vi "drawing fun.vi"() -> ()   [LabVIEW 2009]
panel:
  in  "stop":bool
  out "point":cluster{"x":i16, "y":i16}
  in  "color":u32(colorbox)
  in  "pen":T1={"Width"=1, "Style"=enum."Solid"}
  out "Picture":picture
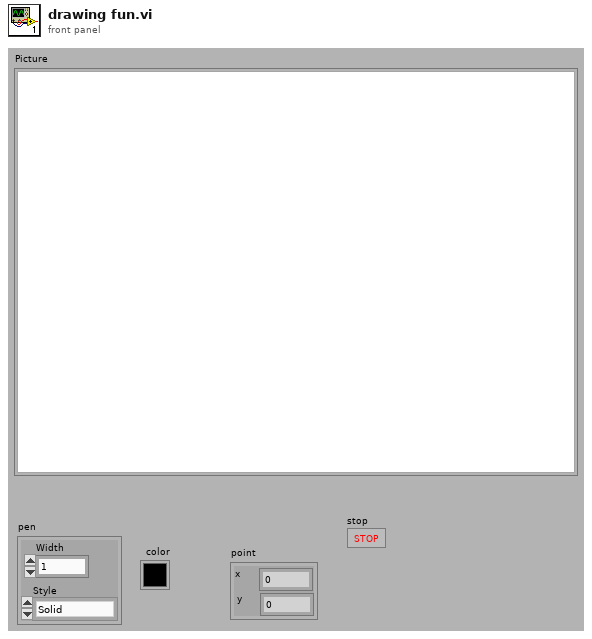
[diagram p1: front panel]
types:
  T1 = cluster{"Width":u16, "Style":enum32{"Solid", "Dash", "Dot", "DashDot", "DashDotDot"}}
  T2 = typedef "LVMouseTypeDef.ctl" = cluster{"Mouse Position":cluster{"X":i32, "Y":i32}, "Mouse Modifiers":cluster{"Button Down":bool, "Shift Mod":bool, "Menu Mod":bool, "Option Mod":bool}}
  T3 = cluster{"Button Down":bool, "Shift Mod":bool, "Menu Mod":bool, "Option Mod":bool}
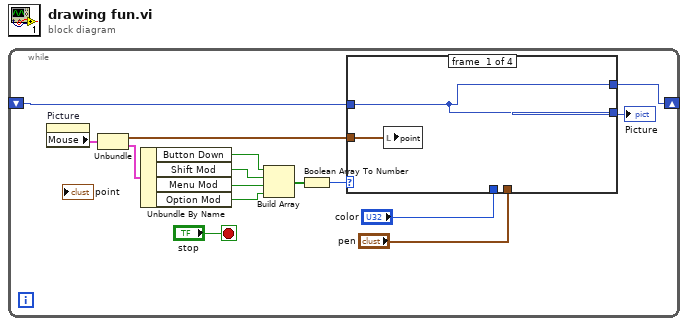
[diagram p0: block diagram]
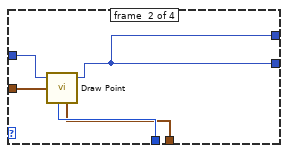
[diagram p2: hidden frame]
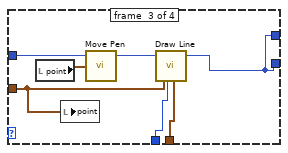
[diagram p3: hidden frame]
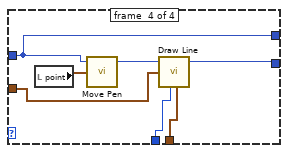
[diagram p4: hidden frame]
diagram:
  n1 = while {
    shift-right: [w2] -> _
    shift-left: _ -> [w3]
    stop <- "stop" stop-if-true
    n2 = property on="Picture" class="Pict"() -> ("Mouse"=w15:T2)  [unwired: 2 in, 2 out]
    n3 = Unbundle(w15) -> ("Mouse Position"=w8:cluster{"X":i32, "Y":i32}, "Mouse Modifiers"=w14:T3)
    n4 = Unbundle By Name(w14) -> ("Button Down"=w5:bool, "Shift Mod"=w13:bool, "Menu Mod"=w12:bool, "Option Mod"=w11:bool)
    n5 = Build Array(w5, w13, w12, w11) -> (w10:bool[])
    n6 = Boolean Array To Number(Boolean array=w10) -> (number=w9:u32)
    n7 = case shown="2" w9 {
      tunnel: w8 -> [w16 w18 w23 w30]
      tunnel: "color" -> [_ w22 w26 w35]
      tunnel: "pen" -> [_ w21 w25 w34]
      tunnel: [w17 w19 w28 w33] -> w4
      tunnel: w3 -> [w17 w20 w29 w32]
      tunnel: [w17 w19 w28 w32] -> w2
      frame #0 {
        n8 = local write "point"(w16) -> ()
      }
      frame #1 {
        n9 = call <vilib>:"Draw Point.vi"("picture"=w20, "point(x,y)"=w18, "color(black)"=w22, "pen"=w21) -> ("new picture"=w19:picture)  [unwired: 5 in]
      }
      frame #2 {
        n10 = local read "point"() -> (w24:cluster{"x":i16, "y":i16})
        n11 = local write "point"(w23) -> ()
        n12 = call <vilib>:"Move Pen.vi"("new position"=w24, "picture"=w29) -> ("new picture"=w27:picture)  [unwired: 3 in]
        n13 = call <vilib>:"Draw Line.vi"("picture"=w27, "end point"=w23, "color(black)"=w26, "pen"=w25) -> ("new picture"=w28:picture)  [unwired: 5 in]
      }
      frame #3 {
        n14 = local read "point"() -> (w31:cluster{"x":i16, "y":i16})
        n15 = call <vilib>:"Move Pen.vi"("new position"=w31, "picture"=w32) -> ("new picture"=w36:picture)  [unwired: 3 in]
        n16 = call <vilib>:"Draw Line.vi"("picture"=w36, "end point"=w30, "color(black)"=w35, "pen"=w34) -> ("new picture"=w33:picture)  [unwired: 5 in]
      }
    }
    "Picture" <- w4
  }
